vi "FTW-JSON-Element-Get.vi"(0 "JSON Opject":string, 5 "Key":string, 11 "error in":errorcluster) -> (8 "Element":string, 10 "Found?":bool, 15 "error out":errorcluster)   [LabVIEW 2015]
uses:
  container/FTW-Container.lvclass
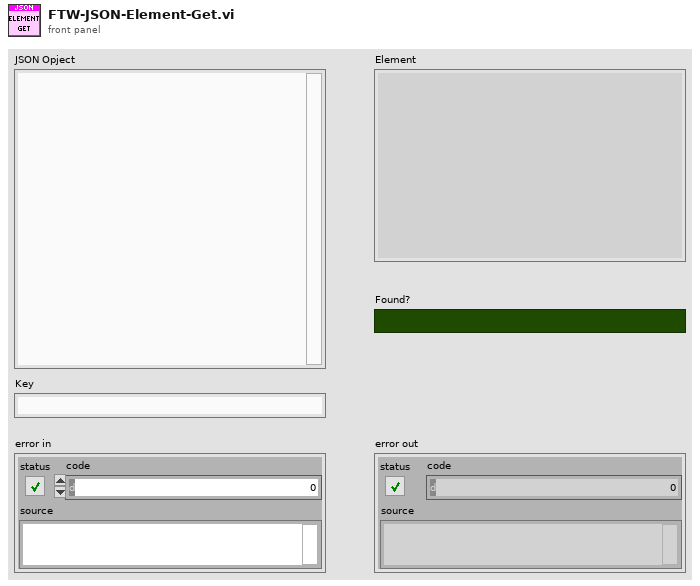
[diagram p1: front panel]
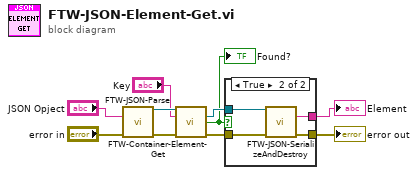
[diagram p0: block diagram]
diagram:
  n1 = call "FTW-JSON-Parse.vi"("JSON String"="JSON Opject", "error in"="error in") -> ("Container"=w6:refnum<class "FTW-Container.lvclass">, "error out"=w9:errorcluster)  [unwired: 12 in]
  n2 = call "FTW-Container-Element-Get.vi"("FTW-Container In"=w6, "Element Name"="Key", "error in"=w9) -> ("Element Out"=w3:refnum<class "FTW-Container.lvclass">, "Found"=w1:bool, "error out"=w7:errorcluster)  [unwired: 9 in, 1 out]
  "Found?" <- w1
  n3 = case shown="True" w1 {
    tunnel: w7 -> [w11 w15]
    tunnel: [w11 w14] -> w4
    tunnel: w3 -> [_ w13]
    tunnel: [_ w12] -> w2
    frame False {
    }
    frame True {
      n4 = call "FTW-JSON-SerializeAndDestroy.vi"("JSON"=w13, "error in"=w15) -> ("JSON String (UTF-8)"=w12:string, "error out"=w14:errorcluster)  [unwired: 12 in]
    }
  }
  "error out" <- w4
  "Element" <- w2
